vi "Software Update HCC Create Version Folder.vi"(8 "Error In":errorcluster, 9 "Software Version":string, 10 "Output Path":path[](array[path]), 11 "Archive Software By Software Type (Ex: C:\\Newfi Exe\\Exe5\\Archive\\Newfi\\)":path) -> (0 "Error Out":errorcluster, 3 "Target Folder":path)   [LabVIEW 2016]
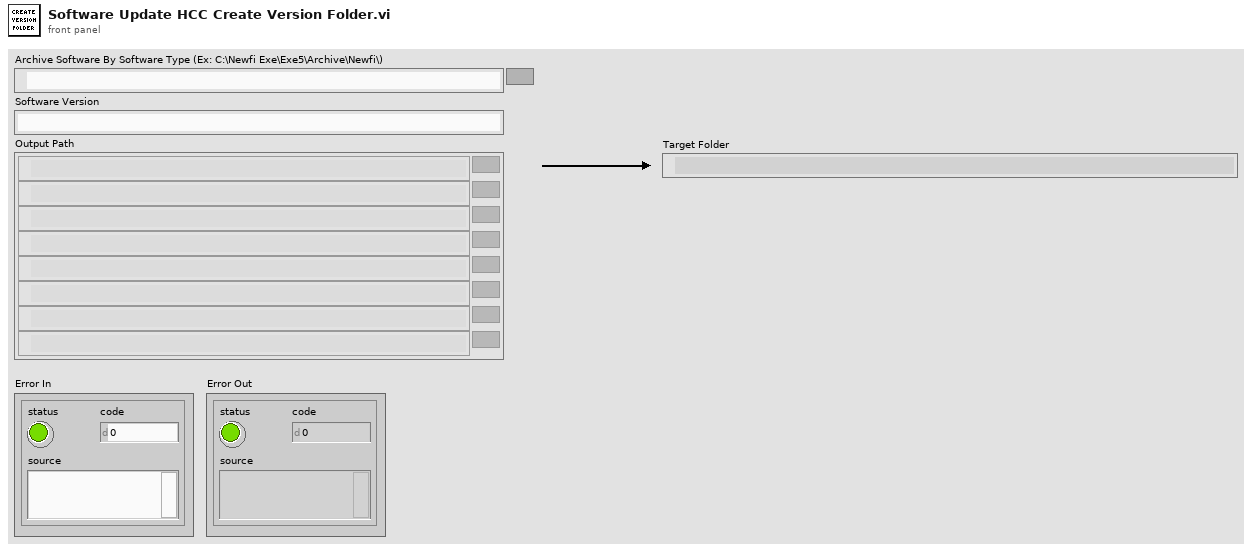
[diagram p1: front panel]
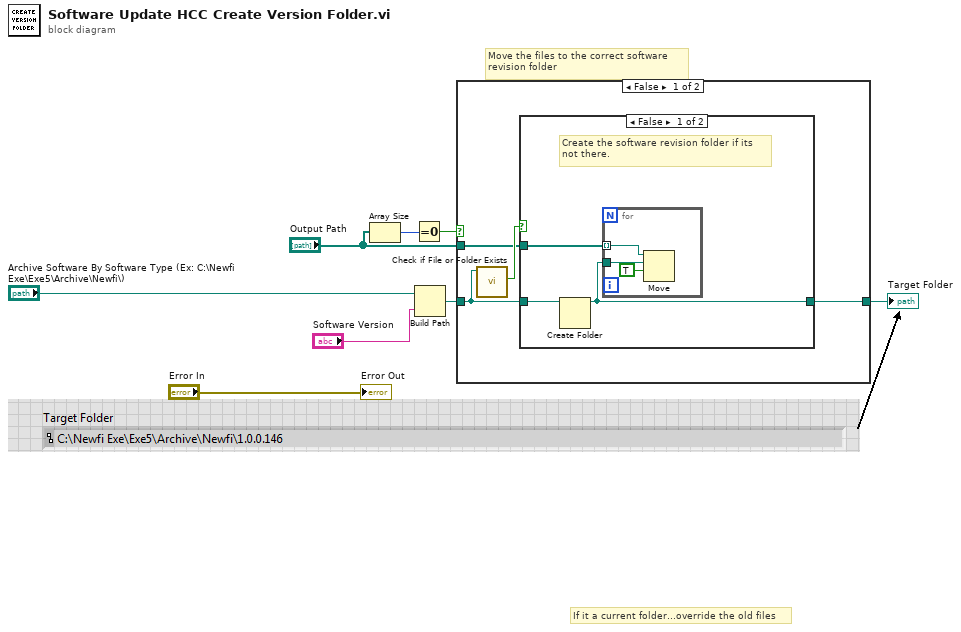
[diagram p0: block diagram]
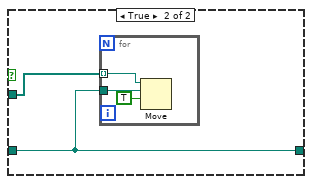
[diagram p2: hidden frame]
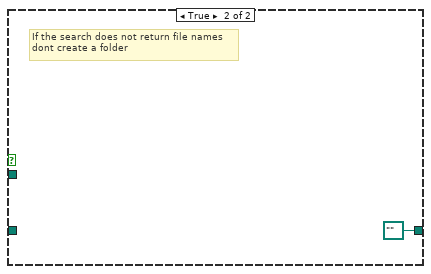
[diagram p3: hidden frame]
diagram:
  # "If it a current folder...override the old files"
  # "Move the files to the correct software \nrevision folder"
  n1 = Array Size(array="Output Path") -> (size(s)=w5:i32)
  n2 = Equal To 0?(x=w5) -> (x = 0?=w6:bool)
  n3 = Build Path(base path="Archive Software By Software Type (Ex: C:\\Newfi Exe\\Exe5\\Archive\\Newfi\\)", name or relative path="Software Version") -> (appended path=w2:path)
  n4 = case shown="False" w6 {
    tunnel: w2 -> [w11 _]
    tunnel: [w10 path "" ("appended path")] -> w3
    tunnel: "Output Path" -> [w9 _]
    frame False {
      n5 = call <vilib>:"Check if File or Folder Exists.vi"("path"=w11) -> ("file or folder exists?"=w12:bool)  [unwired: 8 in, 2 out]
      n6 = case shown="False" w12 {
        tunnel: w11 -> [w15 w19]
        tunnel: w9 -> [w14 w20]
        tunnel: [w13 w19] -> w10
        frame False {
          # "Create the software revision folder if its \nnot there."
          n7 = Create Folder(path (use dialog)=w15) -> (created path=w13:path)  [unwired: 2 in, 2 out]
          n8 = for {
            tunnel: w14 -> [w18] mode=indexing
            tunnel: w13 -> [w17]
            n9 = Move(source path=w18, 9:TRUE ("overwrite (F)"), 10:w17) -> ()  [unwired: 2 in, 3 out]
          }
        }
        frame True {
          n10 = for {
            tunnel: w20 -> [w23] mode=indexing
            tunnel: w19 -> [w22]
            n11 = Move(source path=w23, 9:TRUE ("overwrite (F)"), 10:w22) -> ()  [unwired: 2 in, 3 out]
          }
        }
      }
    }
    frame True {
      # "If the search does not return file names\ndont create a folder"
    }
  }
  "Target Folder" <- w3
  "Error Out" <- "Error In"
